vi "SpeedProtocol.vi"() -> (1 "SpeedProtocol":string, 2 "output 1":i32, 3 "outputProtocol":string)   [LabVIEW 2018]
uses:
  Global Variables.vi
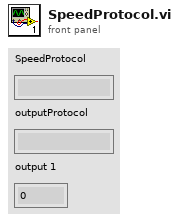
[diagram p1: front panel]
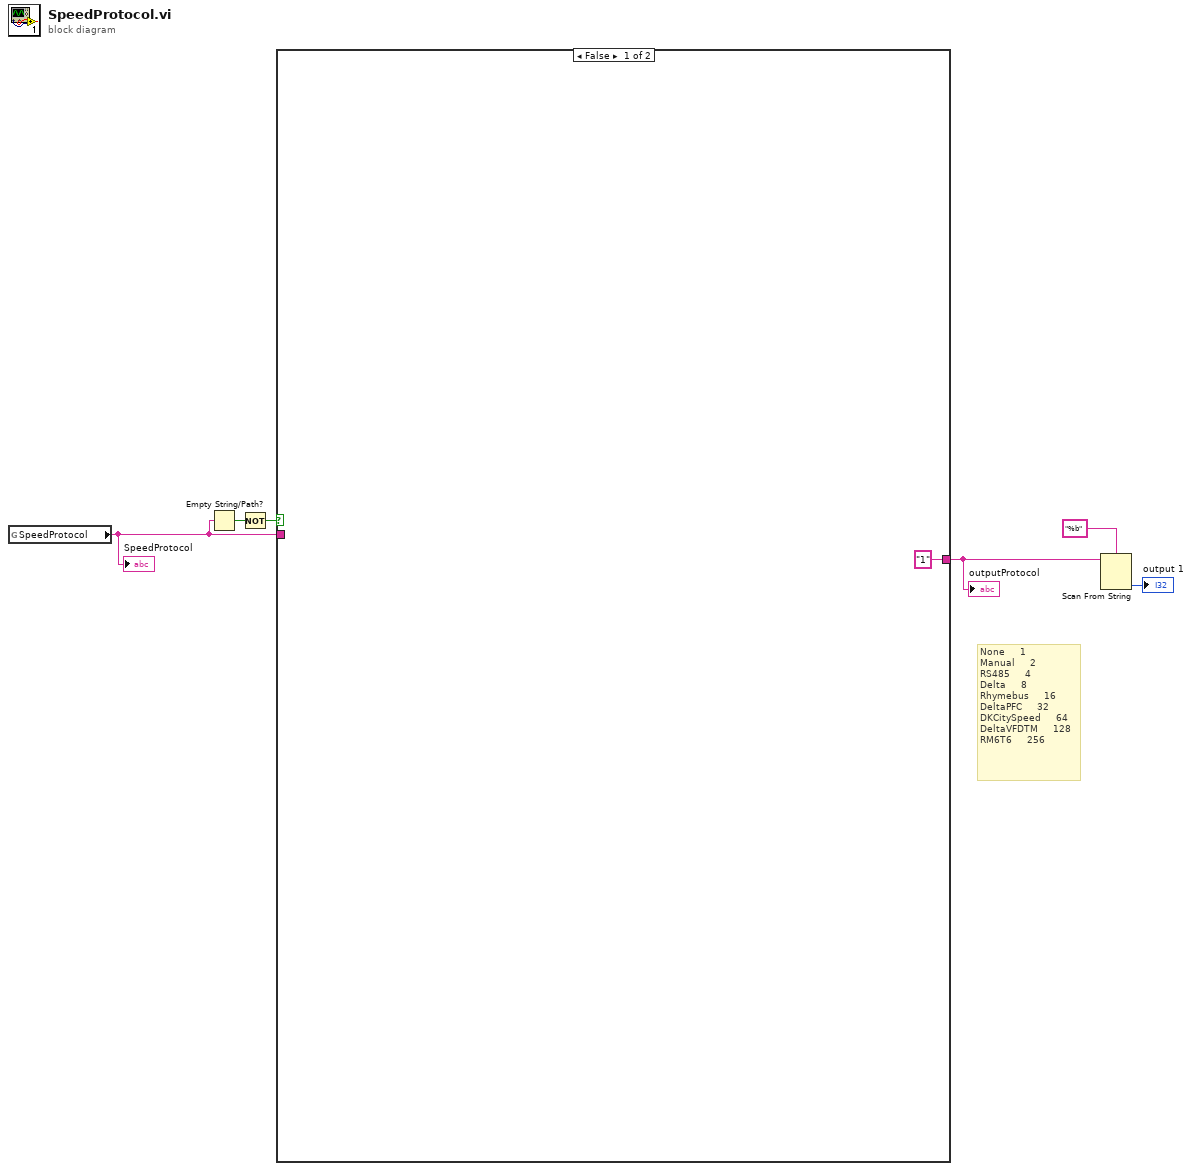
[diagram p0: block diagram]
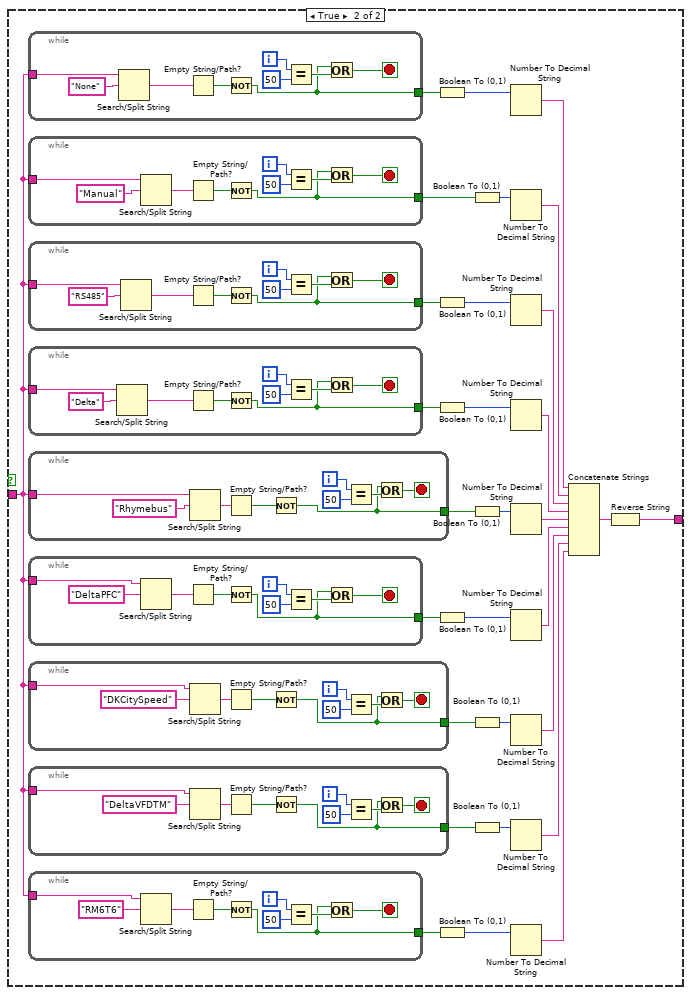
[diagram p2: hidden frame]
diagram:
  # "None     1\nManual     2\nRS485     4\nDelta     8\nRhymebus     16\nDeltaPFC     32\nDKCitySpeed     64\nDeltaVFDTM     128\nRM6T6     256"
  n1 = global read "Global Variables.vi" "SpeedProtocol"() -> (w2:string)
  "SpeedProtocol" <- w2
  n2 = Empty String/Path?(string/path=w2) -> (empty?=w3:bool)
  n3 = Not(x=w3) -> (.not. x?=w1:bool)
  n4 = case shown="False" w1 {
    tunnel: w2 -> [_ w37]
    tunnel: ["1" w8] -> w5
    frame False {
    }
    frame True {
      n5 = while {
        tunnel: w37 -> [w114]
        tunnel: [w110] -> w35
        i -> [w118]
        stop <- w116 stop-if-true
        n6 = Search/Split String(string=w114, search string/char (-)="None") -> (match + rest of string=w111:string)  [unwired: 1 in, 2 out]
        n7 = Empty String/Path?(string/path=w111) -> (empty?=w112:bool)
        n8 = Not(x=w112) -> (.not. x?=w110:bool)
        n9 = Equal?(x=w118, y=50) -> (x = y?=w115:bool)
        n10 = Or(x=w110, y=w115) -> (x .or. y?=w116:bool)
      }
      n11 = while {
        tunnel: w37 -> [w105]
        tunnel: [w101] -> w26
        i -> [w109]
        stop <- w107 stop-if-true
        n12 = Search/Split String(string=w105, search string/char (-)="Manual") -> (match + rest of string=w102:string)  [unwired: 1 in, 2 out]
        n13 = Empty String/Path?(string/path=w102) -> (empty?=w103:bool)
        n14 = Not(x=w103) -> (.not. x?=w101:bool)
        n15 = Equal?(x=w109, y=50) -> (x = y?=w106:bool)
        n16 = Or(x=w101, y=w106) -> (x .or. y?=w107:bool)
      }
      n17 = while {
        tunnel: w37 -> [w96]
        tunnel: [w92] -> w25
        i -> [w100]
        stop <- w98 stop-if-true
        n18 = Search/Split String(string=w96, search string/char (-)="RS485") -> (match + rest of string=w93:string)  [unwired: 1 in, 2 out]
        n19 = Empty String/Path?(string/path=w93) -> (empty?=w94:bool)
        n20 = Not(x=w94) -> (.not. x?=w92:bool)
        n21 = Equal?(x=w100, y=50) -> (x = y?=w97:bool)
        n22 = Or(x=w92, y=w97) -> (x .or. y?=w98:bool)
      }
      n23 = while {
        tunnel: w37 -> [w87]
        tunnel: [w83] -> w24
        i -> [w91]
        stop <- w89 stop-if-true
        n24 = Search/Split String(string=w87, search string/char (-)="Delta") -> (match + rest of string=w84:string)  [unwired: 1 in, 2 out]
        n25 = Empty String/Path?(string/path=w84) -> (empty?=w85:bool)
        n26 = Not(x=w85) -> (.not. x?=w83:bool)
        n27 = Equal?(x=w91, y=50) -> (x = y?=w88:bool)
        n28 = Or(x=w83, y=w88) -> (x .or. y?=w89:bool)
      }
      n29 = while {
        tunnel: w37 -> [w78]
        tunnel: [w74] -> w23
        i -> [w82]
        stop <- w80 stop-if-true
        n30 = Search/Split String(string=w78, search string/char (-)="Rhymebus") -> (match + rest of string=w75:string)  [unwired: 1 in, 2 out]
        n31 = Empty String/Path?(string/path=w75) -> (empty?=w76:bool)
        n32 = Not(x=w76) -> (.not. x?=w74:bool)
        n33 = Equal?(x=w82, y=50) -> (x = y?=w79:bool)
        n34 = Or(x=w74, y=w79) -> (x .or. y?=w80:bool)
      }
      n35 = while {
        tunnel: w37 -> [w69]
        tunnel: [w65] -> w22
        i -> [w73]
        stop <- w71 stop-if-true
        n36 = Search/Split String(string=w69, search string/char (-)="DeltaPFC") -> (match + rest of string=w66:string)  [unwired: 1 in, 2 out]
        n37 = Empty String/Path?(string/path=w66) -> (empty?=w67:bool)
        n38 = Not(x=w67) -> (.not. x?=w65:bool)
        n39 = Equal?(x=w73, y=50) -> (x = y?=w70:bool)
        n40 = Or(x=w65, y=w70) -> (x .or. y?=w71:bool)
      }
      n41 = while {
        tunnel: w37 -> [w60]
        tunnel: [w56] -> w21
        i -> [w64]
        stop <- w62 stop-if-true
        n42 = Search/Split String(string=w60, search string/char (-)="DKCitySpeed") -> (match + rest of string=w57:string)  [unwired: 1 in, 2 out]
        n43 = Empty String/Path?(string/path=w57) -> (empty?=w58:bool)
        n44 = Not(x=w58) -> (.not. x?=w56:bool)
        n45 = Equal?(x=w64, y=50) -> (x = y?=w61:bool)
        n46 = Or(x=w56, y=w61) -> (x .or. y?=w62:bool)
      }
      n47 = while {
        tunnel: w37 -> [w51]
        tunnel: [w47] -> w20
        i -> [w55]
        stop <- w53 stop-if-true
        n48 = Search/Split String(string=w51, search string/char (-)="DeltaVFDTM") -> (match + rest of string=w48:string)  [unwired: 1 in, 2 out]
        n49 = Empty String/Path?(string/path=w48) -> (empty?=w49:bool)
        n50 = Not(x=w49) -> (.not. x?=w47:bool)
        n51 = Equal?(x=w55, y=50) -> (x = y?=w52:bool)
        n52 = Or(x=w47, y=w52) -> (x .or. y?=w53:bool)
      }
      n53 = while {
        tunnel: w37 -> [w42]
        tunnel: [w38] -> w19
        i -> [w46]
        stop <- w44 stop-if-true
        n54 = Search/Split String(string=w42, search string/char (-)="RM6T6") -> (match + rest of string=w39:string)  [unwired: 1 in, 2 out]
        n55 = Empty String/Path?(string/path=w39) -> (empty?=w40:bool)
        n56 = Not(x=w40) -> (.not. x?=w38:bool)
        n57 = Equal?(x=w46, y=50) -> (x = y?=w43:bool)
        n58 = Or(x=w38, y=w43) -> (x .or. y?=w44:bool)
      }
      n59 = Boolean To (0,1)(Boolean=w35) -> (0, 1=w36:i16)
      n60 = Boolean To (0,1)(Boolean=w25) -> (0, 1=w33:i16)
      n61 = Boolean To (0,1)(Boolean=w24) -> (0, 1=w32:i16)
      n62 = Boolean To (0,1)(Boolean=w22) -> (0, 1=w30:i16)
      n63 = Boolean To (0,1)(Boolean=w19) -> (0, 1=w28:i16)
      n64 = Boolean To (0,1)(Boolean=w26) -> (0, 1=w34:i16)
      n65 = Boolean To (0,1)(Boolean=w23) -> (0, 1=w31:i16)
      n66 = Boolean To (0,1)(Boolean=w21) -> (0, 1=w29:i16)
      n67 = Boolean To (0,1)(Boolean=w20) -> (0, 1=w27:i16)
      n68 = Number To Decimal String(number=w36) -> (decimal integer string=w18:string)  [unwired: 1 in]
      n69 = Number To Decimal String(number=w34) -> (decimal integer string=w17:string)  [unwired: 1 in]
      n70 = Number To Decimal String(number=w33) -> (decimal integer string=w16:string)  [unwired: 1 in]
      n71 = Number To Decimal String(number=w32) -> (decimal integer string=w15:string)  [unwired: 1 in]
      n72 = Number To Decimal String(number=w31) -> (decimal integer string=w14:string)  [unwired: 1 in]
      n73 = Number To Decimal String(number=w30) -> (decimal integer string=w13:string)  [unwired: 1 in]
      n74 = Number To Decimal String(number=w29) -> (decimal integer string=w12:string)  [unwired: 1 in]
      n75 = Number To Decimal String(number=w27) -> (decimal integer string=w11:string)  [unwired: 1 in]
      n76 = Number To Decimal String(number=w28) -> (decimal integer string=w10:string)  [unwired: 1 in]
      n77 = Concatenate Strings(w18, w17, w16, w15, w14, w13, w12, w11, w10) -> (w9:string)
      n78 = Reverse String(1:w9) -> (0:w8:string)
    }
  }
  "outputProtocol" <- w5
  n79 = Scan From String(format string="%b", input string=w5) -> (output 1=→"output 1":i32)  [unwired: 3 in, 3 out]
